vi "Example_OE1022 Control.vi"() -> ()   [LabVIEW 2011]
panel:
  out "Freq":dbl
  out "xita":dbl
  out "R":dbl
  in  "Sample count":u32
  in  "Timeout":u32=1000
  in  "Connect":bool
  out "Gain Overlaod":bool
  in  "Remote Mode":u16(ring) items=["USB"=0, "GPIB"=2]
  out "Input Overlaod":bool
  out "PLL Lock":bool
  out "Error":string
  out "Serial Versions":string
  in  "Table":T1(tab) caption="选项卡控件"
  in  "OE1022_Configure Input Filter":T2 {"Input Notch Filter" items=["None"=0, "50Hz"=1, "100Hz"=3, "Both"=2]; "Input Coupling" items=["AC", "DC"]; "Input Shield Grounding" items=["Float", "Ground"]; "Input Source" items=["A", "A-B", "I-1M", "I-100M"]}
  in  "OE1022_Configure Ref Phase":T3={"Reference Source"=0, "Sweep Mode"=0, "Start Frequency"=1000.0, "Stop Frequency"=90000.0, "Linear Step Frequency"=1000.0, "Log Step Percent"=10.0, "Step Time(ms)"=1000, "Sweep Run Mode"=0, "Internal Frequency"=1000.0, "Phase  (degree)"=0.0, "External Ref Trigger"=0} {"External Ref Trigger" items=["TTL Rising Edge", "TTL Falling Edge", "Sine Zero Crossing"]; "Phase  (degree)" min=-180.0 max=180.0 format="%.2f"; "Internal Frequency" min=0.001 max=102000.0 format="%#.3f"; "Sweep Run Mode" items=["Stop", "Singal", "Loop"]; "Step Time(ms)" min=1 max=100000; "Log Step Percent" min=0.0 max=100.0 format="%#.2g"; "Linear Step Frequency" min=0.001 max=102000.0; "Stop Frequency" min=0.001 max=102000.0 format="%#.3f"; "Start Frequency" min=0.001 max=102000.0 format="%#.3f"; "Sweep Mode" items=["Linear", "Log"]; "Reference Source" items=["External", "Internal", "Internal Sweep"]}
  in  "OE1022_Configure Sens and Filter":T4={"Dynamic Reserve"=1, "Sensitivity "=24, "Time Constant "=9, "Low Pass Filter Slope "=1, "Enable Sync Filter "=0} {"Enable Sync Filter" items=["OFF", "ON"]; "Low Pass Filter Slope" items=["6 dB/oct", "12 dB/oct", "18 db/oct", "24 dB/oct"]; "Time Constant" items=["10 us"=1, "30 us"=2, "100 us"=3, "300 us"=4, "1 ms"=5, "3 ms"=6, "10 ms"=7, "30 ms"=8, "100 ms"=9, "300 ms"=10, "1 s"=11, "3 s"=12, "10 s"=13, "30 s"=14, "100 s"=15, "300 s"=16, "1 ks"=17, "3 ks"=18]; "Sensitivity" items=["1 nV/fA"=1, "2 nV/fA"=2, "5 nV/fA"=3, "10 nV/fA"=4, "20 nV/fA"=5, "50 nV/fA"=6, "100 nV/fA"=7, "200 nV/fA"=8, "500 nV/fA"=9, "1 uV/pA"=10, "2 uV/pA"=11, "5 uV/pA"=12, "10 uV/pA"=13, "20 uV/pA"=14, "50 uV/pA"=15, "100 uV/pA"=16, "200 uV/pA"=17, "500 uV/pA"=18, "1 mV/nA"=19, "2 mV/nA"=20, "5 mV/nA"=21, "10 mV/nA"=22, "20 mV/nA"=23, "50 mV/nA"=24, "100 mV/nA"=25, "200 mV/nA"=26, "500 mV/nA"=27, "1 V/uA"=28]; "Dynamic Reserve" items=["Low Noise", "Normal", "High Reserve"]}
  in  "OE1022_Configure Channel Out":T5={"CH1"=0, "CH2"=0, "Speed"=0, "CH2 Offset(%)"=0.0, "CH1 Offset(%)"=0.0, "CH2 Expand"=1, "CH1 Expand"=1} {"CH1 Expand" min=1 max=256; "CH2 Expand" min=1 max=256; "CH1 Offset(%)" min=-100.0 max=100.0 format="%#.2g"; "CH2 Offset(%)" min=-100.0 max=100.0 format="%#.2g"; "Speed" items=["Slow", "Fast"]; "CH2" items=["R", "X", "Y", "Theta", "Rh1", "Xh1", "Yh1", "Theta h1", "Rh2", "Xh2", "Yh2", "Theta h2", "Noise", "E1", "E2", "E3", "E4"]; "CH1" items=["R", "X", "Y", "Theta", "Rh1", "Xh1", "Yh1", "Theta h1", "Rh2", "Xh2", "Yh2", "Theta h2", "Noise", "E1", "E2", "E3", "E4"]}
  in  "OE1022_Configure Sine Out":T6={"Start Value(V)"=0.1, "Sine Output Amplitude (V)"=0.1, "Stop Valve(V)"=1.0, "Sine Step Valve(V)"=0.1, "Step Time(ms) "=1000, "Sine Step Percent(%)"=10.0, "SineOut Mode"=0, "Sine Run Mode"=0} {"Sine Run Mode" items=["Stop", "Single", "Loop"]; "SineOut Mode" items=["Fixed", "Linear", "Log"]; "Sine Step Percent(%)" min=0.0 max=100.0 format="%#.3g"; "Step Time(ms)" min=1 max=100000; "Sine Step Valve(V)" min=0.001 max=5.0 format="%#.3g"; "Stop Valve(V)" min=0.0001 max=5.0 format="%#.3g"; "Sine Output Amplitude (V)" min=0.0001 max=5.0 format="%#.3g"; "Start Value(V)" min=0.001 max=5.0 format="%#.3g"}
  in  "OE1022_Configure Harmonic":cluster{"Harmonic 1":u16, "Harmonic 2":u16}={"Harmonic 1"=1, "Harmonic 2"=1} {"Harmonic 2" min=1 max=32767; "Harmonic 1" min=1 max=32767}
  in  "OE1022_Configure DAC":T7 {"DAC4 Output" min=-10.0 max=10.0 format="%#_4g"; "DAC3 Output" min=-10.0 max=10.0 format="%#_4g"; "DAC2 Output" min=-10.0 max=10.0 format="%#_4g"; "DAC1 Output" min=-10.0 max=10.0 format="%#_4g"}
  in  "OE1022_Configure Sample":T8={"Trigger Mode"=0, "Sample Mode"=0, "Buffer 1"=0, "Buffer 2"=1, "Buffer 3"=2, "Sample Time(ms)"=100, "Length"=50, "Buffer 4"=3, "Sample State"=2} {"Sample State" items=["Start", "Pause", "Stop and Clear"]; "Buffer 4" items=["R", "X", "Y", "Theta", "Rh1", "Xh1", "Yh1", "Theta h1", "Rh2", "Xh2", "Yh2", "Theta h2", "Noise", "A1", "A2", "A3", "A4", "Freq", "C1", "C2"]; "Length" min=1 max=16384; "Sample Time(ms)" min=1 max=100000; "Buffer 3" items=["R", "X", "Y", "Theta", "Rh1", "Xh1", "Yh1", "Theta h1", "Rh2", "Xh2", "Yh2", "Theta h2", "Noise", "A1", "A2", "A3", "A4", "Freq", "C1", "C2"]; "Buffer 2" items=["R", "X", "Y", "Theta", "Rh1", "Xh1", "Yh1", "Theta h1", "Rh2", "Xh2", "Yh2", "Theta h2", "Noise", "A1", "A2", "A3", "A4", "Freq", "C1", "C2"]; "Buffer 1" items=["R", "X", "Y", "Theta", "Rh1", "Xh1", "Yh1", "Theta h1", "Rh2", "Xh2", "Yh2", "Theta h2", "Noise", "A1", "A2", "A3", "A4", "Freq", "C1", "C2"]; "Sample Mode" items=["Single", "Loop"]; "Trigger Mode" items=["Int", "Ext"]}
  in  "Save Button":bool
  in  "file path":path
  in  "Sample Rate":dbl=0.1 min=0.1 max=100.0
  in  "OE1022_Configure Equation":T9={"A"=0, "B"=18, "C"=19, "E"=1, "C1"=0.0, "C2"=0.0} {"C2" min=-10.0 max=10.0 format="%.3f"; "C1" min=-10.0 max=10.0 format="%.3f"; "E" items=["1"=1, "2"=2, "3"=3, "4"=4]; "C" items=["R", "X", "Y", "Theta", "Rh1", "Xh1", "Yh1", "Theta h1", "Rh2", "Xh2", "Yh2", "Theta h2", "Noise", "A1", "A2", "A3", "A4", "Freq", "C1", "C2"]; "B" items=["R", "X", "Y", "Theta", "Rh1", "Xh1", "Yh1", "Theta h1", "Rh2", "Xh2", "Yh2", "Theta h2", "Noise", "A1", "A2", "A3", "A4", "Freq", "C1", "C2"]; "A" items=["R", "X", "Y", "Theta", "Rh1", "Xh1", "Yh1", "Theta h1", "Rh2", "Xh2", "Yh2", "Theta h2", "Noise", "A1", "A2", "A3", "A4", "Freq", "C1", "C2"]}
  in  "OE1022_Auto Setting":T10
  out "Status":string
  in  "VISA resource name":refnum<visa-resource-name>
  in  "Baud Rate (921600)":u32=921600
  # "Tel          :   +86-020-84133345\nWebsite  :   www.ssi-instrument.com\nE-mail     :   support@si-instrument.com"
  # "X"
  # "="
  # "______________________________________________________"
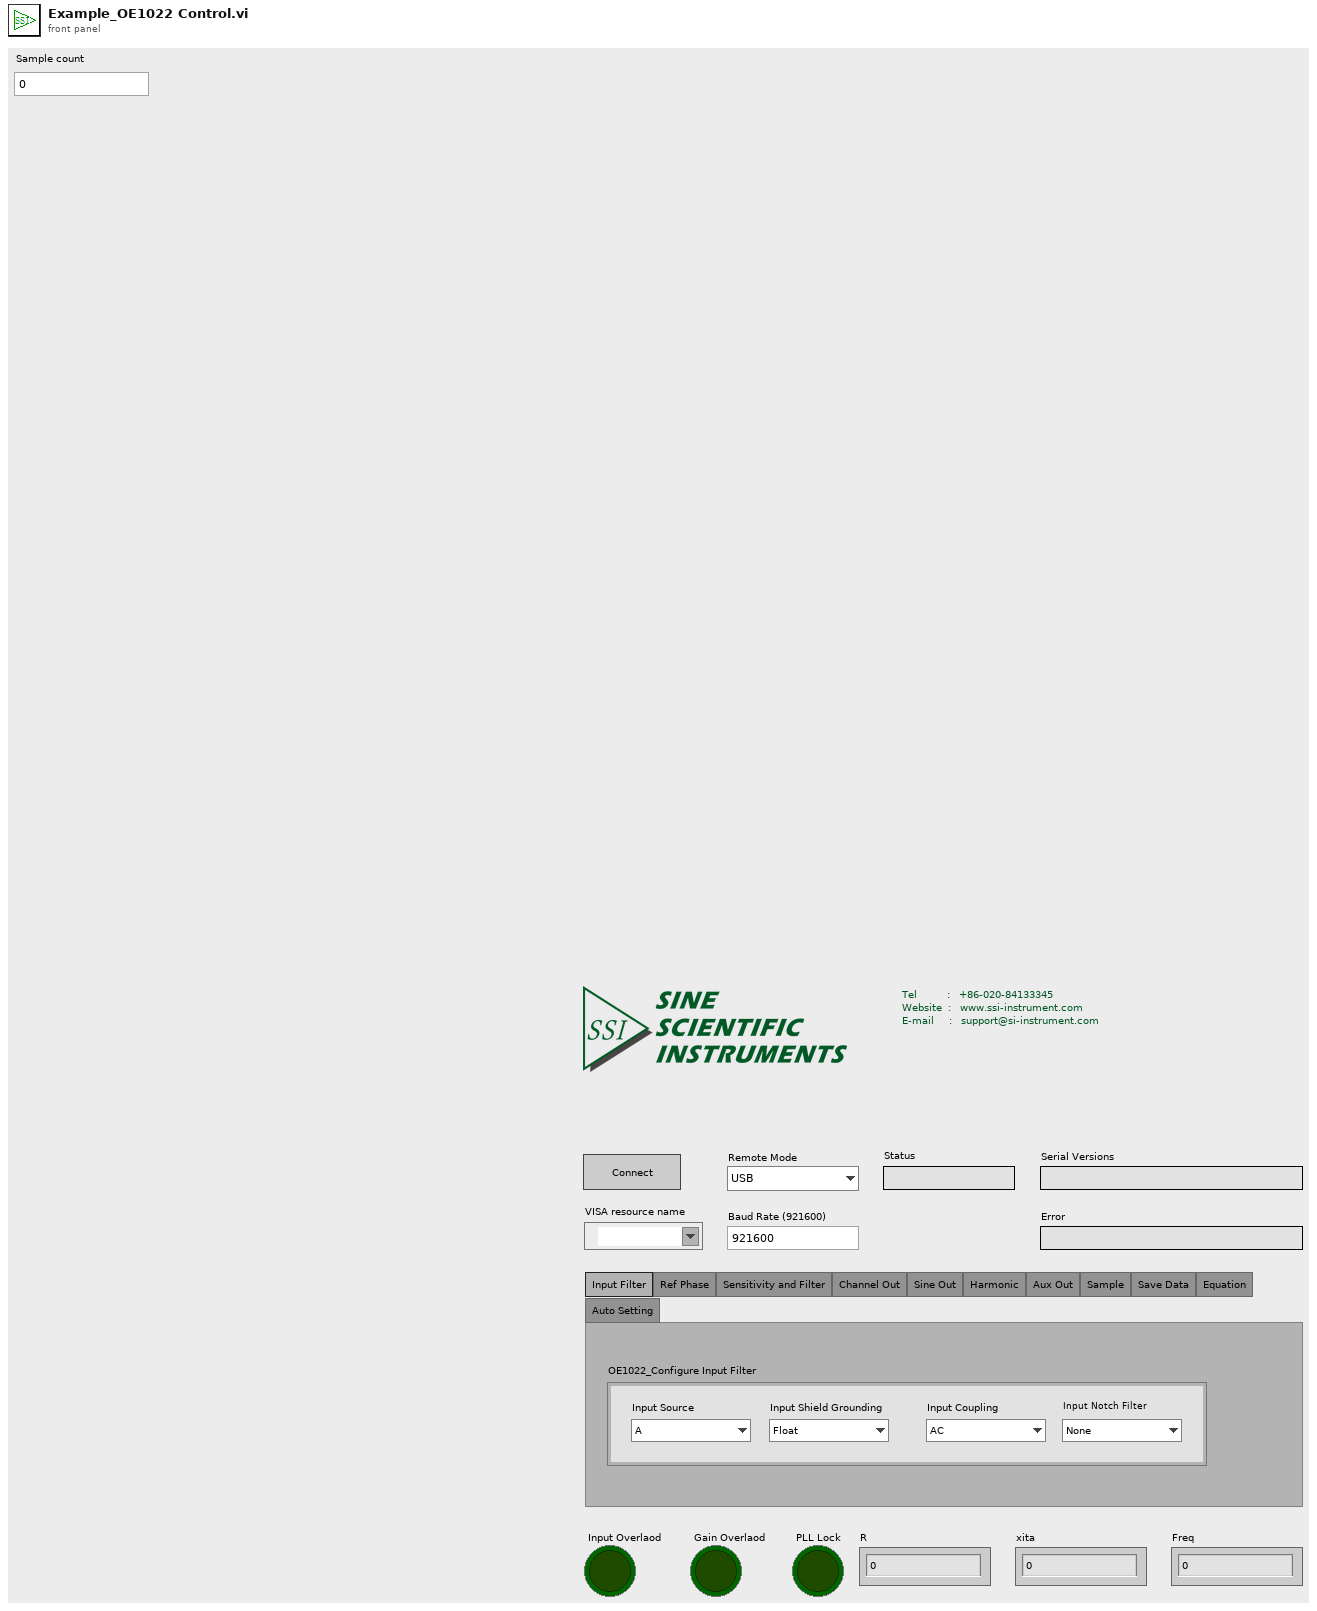
[diagram p1: front panel]
types:
  T1 = enum32{"Input Filter", "Ref Phase", "Sensitivity and Filter", "Channel Out", "Sine Out", "Harmonic", "Aux Out", "Sample", "Save Data", "Equation", "Auto Setting"}
  T2 = cluster{"Input Source":u16, "Input Shield Grounding ":u16, "Input Coupling ":u16, "Input Notch Filter ":u16}
  T3 = cluster{"Reference Source":u16, "Sweep Mode":u16, "Start Frequency":dbl, "Stop Frequency":dbl, "Linear Step Frequency":dbl, "Log Step Percent":dbl, "Step Time(ms)":i32, "Sweep Run Mode":u16, "Internal Frequency":dbl, "Phase  (degree)":dbl, "External Ref Trigger":u16}
  T4 = cluster{"Dynamic Reserve":u16, "Sensitivity ":u16, "Time Constant ":u8, "Low Pass Filter Slope ":u8, "Enable Sync Filter ":u16}
  T5 = cluster{"CH1":u16, "CH2":u16, "Speed":u16, "CH2 Offset(%)":dbl, "CH1 Offset(%)":dbl, "CH2 Expand":i16, "CH1 Expand":i16}
  T6 = cluster{"Start Value(V)":dbl, "Sine Output Amplitude (V)":dbl, "Stop Valve(V)":dbl, "Sine Step Valve(V)":dbl, "Step Time(ms) ":u32, "Sine Step Percent(%)":dbl, "SineOut Mode":u8, "Sine Run Mode":u8}
  T7 = cluster{"DAC1 Output":dbl, "DAC2 Output":dbl, "DAC3 Output":dbl, "DAC4 Output":dbl}
  T8 = cluster{"Trigger Mode":u16, "Sample Mode":u16, "Buffer 1":u16, "Buffer 2":u16, "Buffer 3":u16, "Sample Time(ms)":u32, "Length":u16, "Buffer 4":u16, "Sample State":u16}
  T9 = cluster{"A":u16, "B":u16, "C":u16, "E":u16, "C1":dbl, "C2":dbl}
  T10 = cluster{"Auto Gain":bool, "Auto Reserve":bool, "Auto Phase":bool, "Auto Scale":bool}
  T11 = enum16{"OE1022", "OE1022D", "OE1201", "OE2031&OE2041", "OE1311&OE1351"}
  T12 = cluster{"PLL Lock(1: External Lock)":bool, "Input Overlaod":bool, "Gain Overlaod":bool}
  T13 = cluster{"X":dbl, "Y":dbl, "R":dbl, "θ":dbl, "Frequency":dbl, "Xh1":dbl, "Yh1":dbl, "Rh1":dbl, "θh1":dbl, "Xh2":dbl, "Yh2":dbl, "Rh2":dbl, "θh2":dbl, "Noise":dbl, "A1":dbl, "A2":dbl, "A3":dbl, "A4":dbl}
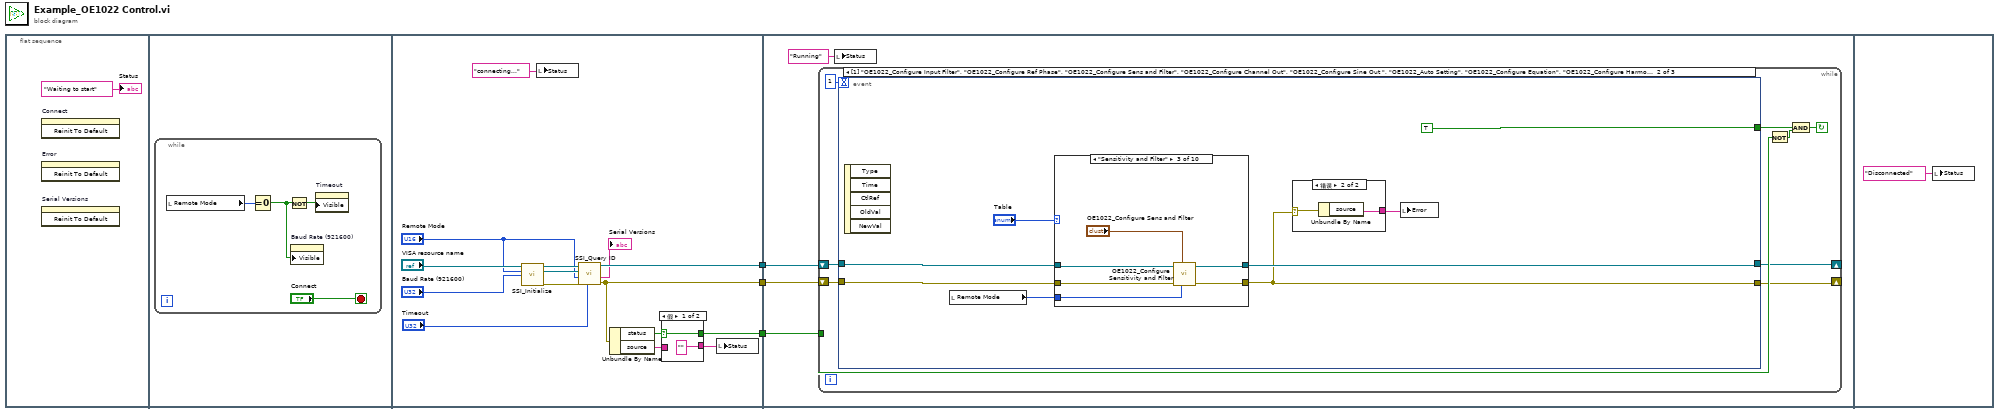
[diagram p0: block diagram]
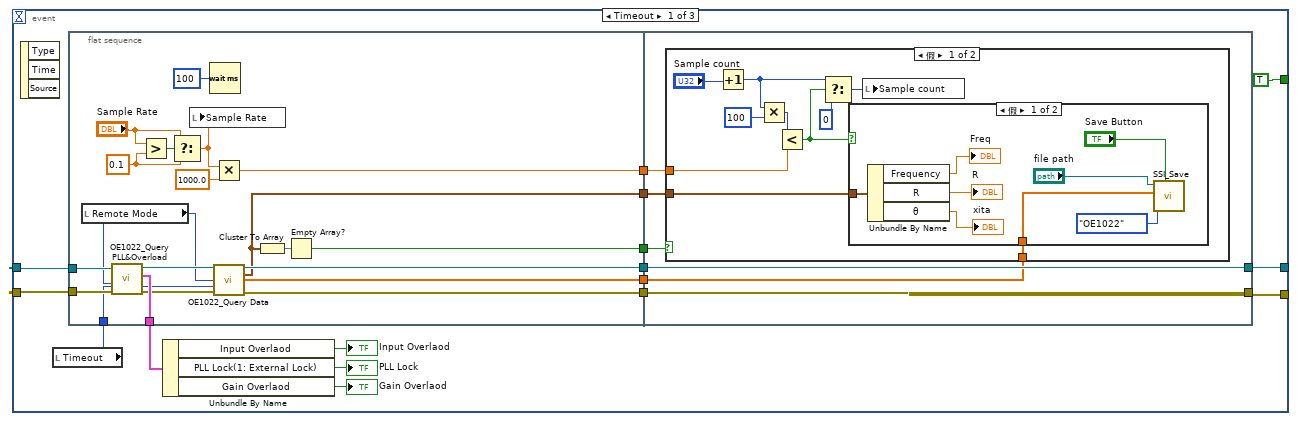
[diagram p3: hidden frame]
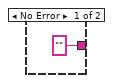
[diagram p6: hidden frame]
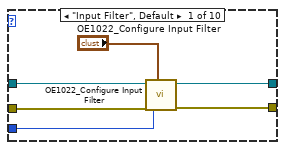
[diagram p7: hidden frame]
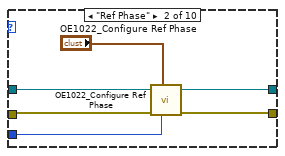
[diagram p8: hidden frame]
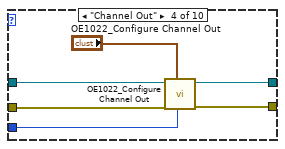
[diagram p9: hidden frame]
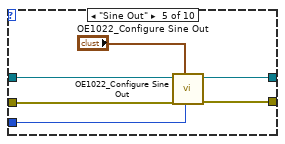
[diagram p10: hidden frame]
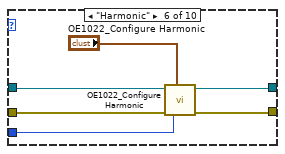
[diagram p11: hidden frame]
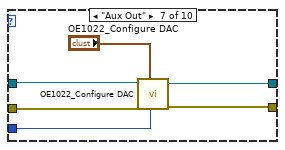
[diagram p12: hidden frame]
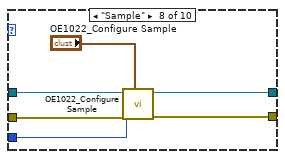
[diagram p13: hidden frame]
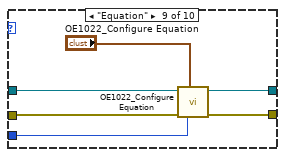
[diagram p14: hidden frame]
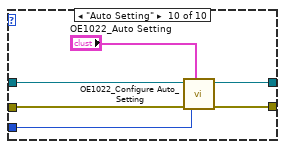
[diagram p15: hidden frame]
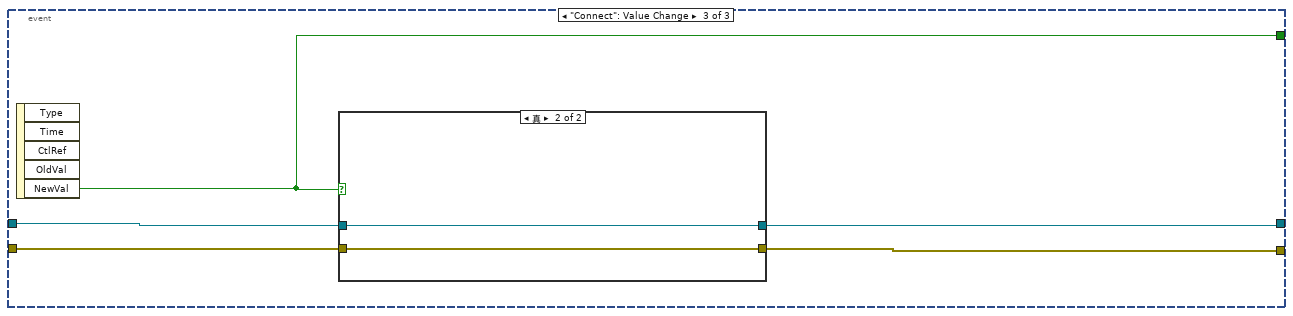
[diagram p16: hidden frame]
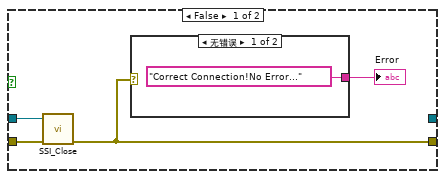
[diagram p17: hidden frame]
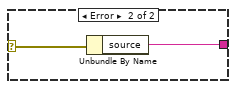
[diagram p18: hidden frame]
diagram:
  n1 = flat-sequence {
    tunnel: [w17] -> w3
    tunnel: [w14] -> w2
    tunnel: [w12] -> w1
    tunnel: w3 -> [w30]
    tunnel: w2 -> [w29]
    tunnel: w1 -> [w28]
    frame #0 {
      n2 = invoke on="Connect" class="Bool (严格)" method="Reinit To Default"() -> ()  [unwired: 3 in, 3 out]
      n3 = invoke on="Error" class="Str" method="Reinit To Default"() -> ()  [unwired: 3 in, 3 out]
      n4 = invoke on="Serial Versions" class="Str" method="Reinit To Default"() -> ()  [unwired: 3 in, 3 out]
      "Status" <- "Waiting to start" ("status")
    }
    frame #1 {
      n5 = while {
        stop <- "Connect" stop-if-true
        n6 = local read "Remote Mode"() -> (w7:u16)
        n7 = Equal To 0?(x=w7) -> (x = 0?=w5:bool)
        n8 = Not(x=w5) -> (.not. x?=w6:bool)
        n9 = property on="Baud Rate (921600)" class="DigNum (严格)"("Visible"=w5) -> ()  [unwired: 2 in, 2 out]
        n10 = property on="Timeout" class="DigNum (严格)"("Visible"=w6) -> ()  [unwired: 2 in, 2 out]
      }
    }
    frame #2 {
      n11 = call "SSI_Initialize.vi"("VISA resource name"="VISA resource name", "Remote Mode"="Remote Mode", "baud rate (921600)"="Baud Rate (921600)") -> ("VISA resource name out"=w21:refnum<visa-resource-name>, "connection ID(Ethernet)"=w20:refnum<k5>, "error out"=w19:errorcluster)  [unwired: 10 in]
      n12 = local write "Status"("connecting..." ("status")) -> ()
      n13 = call "SSI_Query ID.vi"("Timeout"="Timeout", "Error in (no error)"=w19, "Remote Mode"="Remote Mode", "Connection ID in"=w20, "VISA resource name"=w21) -> ("Error out"=w14:errorcluster, "Read Buffer"=→"Serial Versions":string, "VISA resource  out"=w17:refnum<visa-resource-name>)  [unwired: 3 in, 1 out]
      n14 = Unbundle By Name(w14) -> ("status"=w13:bool, "source"=w10:string)
      n15 = case shown="假" w13 {
        selector: w13 -> [w25 w27]
        tunnel: [w25 w27] -> w12
        tunnel: ["" w26] -> w11
        tunnel: w10 -> [_ w26]
        frame False {
        }
        frame True {
        }
      }
      n16 = local write "Status"(w11) -> ()
    }
    frame #3 {
      n17 = while {
        tunnel: w28 -> [w36]
        shift-right: [w33] -> _
        shift-left: w30 -> [w35]
        shift-right: [w32] -> _
        shift-left: w29 -> [w34]
        stop <- w38 continue-if-true
        n18 = event shown="[1] \"OE1022_Configure Input Filter\", \"OE1022_Configure Ref Phase\", \"OE1022_Configure Sens and Filter\", \"OE1022_Configure Channel Out\", \"OE1022_Configure Sine Out \", \"OE1022_Auto Setting\", \"OE1022_Configure Equation\", \"OE1022_Configure Harmonic \", \"OE1022_Configure DAC\", \"OE1022_Configure Sample\": 值改变" {
          selector: _ -> [_ _ _]
          dyn-events: _ -> [_ _ _]
          timeout: 1 -> [_ _ _]
          tunnel: [TRUE ("Stop") TRUE ("Stop") w172] -> w37
          tunnel: [w52 w101 w174] -> w32
          tunnel: [w53 w105 w173] -> w33
          tunnel: w35 -> [w55 w107 w176]
          tunnel: w34 -> [w54 w106 w175]
          event Timeout {
            n19 = event-data() -> ()  [unwired: 1 in, 3 out]
            n20 = local read "Timeout"() -> (w41:u32)
            n21 = flat-sequence {
              tunnel: [w57] -> w47
              tunnel: [w68] -> w46
              tunnel: [w71] -> w45
              tunnel: [w70] -> w44
              tunnel: [w67] -> w43
              tunnel: [w66] -> w42
              tunnel: [w65] -> w51
              tunnel: w55 -> [w63]
              tunnel: w54 -> [w62]
              tunnel: w41 -> [w60]
              tunnel: w47 -> [w81]
              tunnel: w46 -> [w82]
              tunnel: [w82] -> w53
              tunnel: [w81] -> w52
              tunnel: w45 -> [w78]
              tunnel: w44 -> [w77]
              tunnel: w43 -> [w79]
              tunnel: w42 -> [w80]
              frame #0 {
                w74 = 0.1 ("y")
                n22 = local read "Remote Mode"() -> (w59:u16)
                n23 = call "OE1022_Query PLL&Overload.vi"("Timeout"=w60, "Error in (no error)"=w62, "Remote Mode"=w59, "VISA resource name"=w63) -> ("Error out"=w58:errorcluster, "OE1022_Query PLL&Overload"=w65:T12, "VISA resource  out"=w69:refnum<visa-resource-name>)  [unwired: 4 in, 1 out]
                n24 = Greater?(x="Sample Rate", y=w74) -> (0:w73:bool)
                n25 = Select(t="Sample Rate", s=w73, f=w74) -> (s? t:f=w72:dbl)
                n26 = local write "Sample Rate"(w72) -> ()
                n27 = Wait (ms)(milliseconds to wait=u32 100 ("等待时间（毫秒）")) -> ()  [unwired: 1 out]
                n28 = Multiply(x=w72, y=1000.0) -> (x*y=w70:dbl)
                n29 = call "OE1022_Query Data.vi"("VISA resource name"=w69, "Remote Mode"=w59, "Timeout"=w60, "Error in (no error)"=w58) -> ("VISA resource  out"=w68:refnum<visa-resource-name>, "Parameter Values"=w67:T13, "Data Array"=w66:dbl[], "Error out"=w57:errorcluster)  [unwired: 7 in, 1 out]
                n30 = Cluster To Array(cluster=w67) -> (array=w76:dbl[])
                n31 = Empty Array?(array=w76) -> (empty?=w71:bool)
              }
              frame #1 {
                n32 = case shown="假" w78 {
                  tunnel: w80 -> [w92 _]
                  tunnel: w79 -> [w91 _]
                  tunnel: w77 -> [w88 _]
                  frame False {
                    n33 = Increment(x="Sample count") -> (x+1=w85:u32)
                    n34 = Multiply(x=w85, y=u32 100) -> (x*y=w89:u32)
                    n35 = Less?(x=w89, y=w88) -> (x < y?=w86:bool)
                    n36 = Select(t=w85, s=w86, f=0) -> (s? t:f=w84:u32)
                    n37 = case shown="假" w86 {
                      tunnel: w91 -> [w100 _]
                      tunnel: w92 -> [w99 _]
                      frame False {
                        n38 = Unbundle By Name(w100) -> ("Frequency"=→"Freq":dbl, "R"=→"R":dbl, "θ"=→"xita":dbl)
                        n39 = call "SSI_Save.vi"("file path (dialog if empty)"="file path", "1D data"=w99, "Instrument Mode"=T11."OE1022", "Save Button"="Save Button") -> ()  [unwired: 7 in]
                      }
                      frame True {
                      }
                    }
                    n40 = local write "Sample count"(w84) -> ()
                  }
                  frame True {
                  }
                }
              }
            }
            n41 = Unbundle By Name(w51) -> ("Input Overlaod"=→"Input Overlaod":bool, "PLL Lock(1: External Lock)"=→"PLL Lock":bool, "Gain Overlaod"=→"Gain Overlaod":bool)
          }
          event "OE1022_Configure Input Filter", "OE1022_Configure Ref Phase", "OE1022_Configure Sens and Filter", "OE1022_Configure Channel Out", "OE1022_Configure Sine Out", "OE1022_Auto Setting", "OE1022_Configure Equation", "OE1022_Configure Harmonic", "OE1022_Configure DAC", "OE1022_Configure Sample": Value Change {
            n42 = event-data() -> ()  [unwired: 1 in, 5 out]
            n43 = local read "Remote Mode"() -> (w103:u16)
            n44 = case shown="\"Sensitivity and Filter\"" "Table" {
              tunnel: w107 -> [w117 w123 w126 w133 w139 w146 w149 w158 w162 w168]
              tunnel: w106 -> [w116 w122 w129 w135 w141 w147 w152 w159 w163 w169]
              tunnel: [w114 w120 w127 w132 w138 w145 w150 w155 w165 w171] -> w105
              tunnel: [w115 w121 w128 w134 w140 w144 w151 w156 w164 w170] -> w101
              tunnel: w103 -> [w112 w119 w125 w130 w136 w142 w148 w157 w161 w167]
              frame "Input Filter", Default {
                n45 = call "OE1022_Configure Input Filter.vi"("OE1022_Configure Input Filter"="OE1022_Configure Input Filter", "Error in (no error)"=w116, "Remote Mode"=w112, "VISA resource name"=w117) -> ("Error out"=w115:errorcluster, "VISA resource  out"=w114:refnum<visa-resource-name>)  [unwired: 5 in, 1 out]
              }
              frame "Ref Phase" {
                n46 = call "OE1022_Configure Ref Phase.vi"("OE1022_Configure Ref Phase"="OE1022_Configure Ref Phase", "Error in (no error)"=w122, "Remote Mode"=w119, "VISA resource name"=w123) -> ("Error out"=w121:errorcluster, "VISA resource  out"=w120:refnum<visa-resource-name>)  [unwired: 5 in, 1 out]
              }
              frame "Sensitivity and Filter" {
                n47 = call "OE1022_Configure Sensitivity and Filter.vi"("OE1022_Configure Sens and Filter"="OE1022_Configure Sens and Filter", "Error in (no error)"=w129, "Remote Mode"=w125, "VISA resource name"=w126) -> ("Error out"=w128:errorcluster, "VISA resource  out"=w127:refnum<visa-resource-name>)  [unwired: 5 in, 1 out]
              }
              frame "Channel Out" {
                n48 = call "OE1022_Configure Channel Out.vi"("OE1022_Configure Channel Out"="OE1022_Configure Channel Out", "Error in (no error)"=w135, "Remote Mode"=w130, "VISA resource name"=w133) -> ("Error out"=w134:errorcluster, "VISA resource  out"=w132:refnum<visa-resource-name>)  [unwired: 5 in, 1 out]
              }
              frame "Sine Out" {
                n49 = call "OE1022_Configure Sine Out.vi"("OE1022_Configure Sine Out"="OE1022_Configure Sine Out", "Error in (no error)"=w141, "Remote Mode"=w136, "VISA resource name"=w139) -> ("Error out"=w140:errorcluster, "VISA resource  out"=w138:refnum<visa-resource-name>)  [unwired: 5 in, 1 out]
              }
              frame "Harmonic" {
                n50 = call "OE1022_Configure Harmonic.vi"("OE1022_Configure Harmonic"="OE1022_Configure Harmonic", "Error in (no error)"=w147, "Remote Mode"=w142, "VISA resource name"=w146) -> ("Error out"=w144:errorcluster, "VISA resource  out"=w145:refnum<visa-resource-name>)  [unwired: 5 in, 1 out]
              }
              frame "Aux Out" {
                n51 = call "OE1022_Configure DAC.vi"("OE1022_Configure DAC"="OE1022_Configure DAC", "Error in (no error)"=w152, "Remote Mode"=w148, "VISA resource name"=w149) -> ("Error out"=w151:errorcluster, "VISA resource  out"=w150:refnum<visa-resource-name>)  [unwired: 5 in, 1 out]
              }
              frame "Sample" {
                n52 = call "OE1022_Configure Sample.vi"("OE1022_Configure Sample"="OE1022_Configure Sample", "Error in (no error)"=w159, "Remote Mode"=w157, "VISA resource name"=w158) -> ("Error out"=w156:errorcluster, "VISA resource  out"=w155:refnum<visa-resource-name>)  [unwired: 5 in, 1 out]
              }
              frame "Equation" {
                n53 = call "OE1022_Configure Equation.vi"("OE1022_Configure Equation"="OE1022_Configure Equation", "Error in (no error)"=w163, "Remote Mode"=w161, "VISA resource name"=w162) -> ("Error out"=w164:errorcluster, "VISA resource  out"=w165:refnum<visa-resource-name>)  [unwired: 5 in, 1 out]
              }
              frame "Auto Setting" {
                n54 = call "OE1022_Configure Auto_Setting.vi"("OE1022_Auto Setting"="OE1022_Auto Setting", "Error in (no error)"=w169, "Remote Mode"=w167, "VISA resource name"=w168) -> ("Error out"=w170:errorcluster, "VISA resource  out"=w171:refnum<visa-resource-name>)  [unwired: 5 in, 1 out]
              }
            }
            n55 = case shown="错误" w101 {
              selector: w101 -> [_ w111]
              tunnel: ["" ("source") w110] -> w102
              frame No Error {
              }
              frame Error {
                n56 = Unbundle By Name(w111) -> ("source"=w110:string)
              }
            }
            n57 = local write "Error"(w102) -> ()
          }
          event "Connect": Value Change {
            n58 = event-data() -> ("NewVal"=w172:bool)  [unwired: 1 in, 4 out]
            n59 = case shown="真" w172 {
              tunnel: w176 -> [w180 w184]
              tunnel: w175 -> [w179 w185]
              tunnel: [w178 w185] -> w174
              tunnel: [_ w184] -> w173
              frame False {
                n60 = call "SSI_Close.vi"("Error in (no error)"=w179, "VISA resource name"=w180) -> ("Error out"=w178:errorcluster)  [unwired: 5 in]
                n61 = case shown="无错误" w178 {
                  selector: w178 -> [_ w183]
                  tunnel: ["Correct Connection!No Error..." ("source") w182] -> w177
                  frame No Error {
                  }
                  frame Error {
                    n62 = Unbundle By Name(w183) -> ("source"=w182:string)
                  }
                }
                "Error" <- w177
              }
              frame True {
              }
            }
          }
        }
        n63 = Not(x=w36) -> (.not. x?=w39:bool)
        n64 = And(x=w37, y=w39) -> (x .and. y?=w38:bool)
      }
      n65 = local write "Status"("Running" ("status")) -> ()
    }
    frame #4 {
      n66 = local write "Status"("Disconnected" ("status")) -> ()
    }
  }
